vi "createArrayTriggIdx.vi"(1 "CTO parameter ID":i32[](array[numeric])=[2, 3, 1, 10, 9], 2 "triggOutputIdx":string) -> (0 "Array":string[](array[string]))   [LabVIEW 2015]
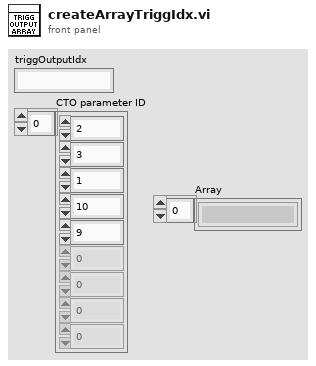
[diagram p1: front panel]
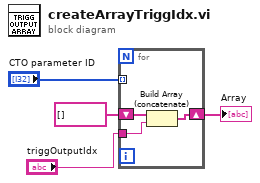
[diagram p0: block diagram]
diagram:
  n1 = for {
    shift-right: [w5] -> w1
    shift-left: string[] [] -> [w7]
    tunnel: "triggOutputIdx" -> [w6]
    tunnel: "CTO parameter ID" -> [_] mode=indexing
    n2 = Build Array (concatenate)(w7, w6) -> (w5:string[])
  }
  "Array" <- w1
